vi "FTW-Tag-Core_Initialize.vi"(0 "Initialization Sequence":string, 5 "FTW Actor Instance Configuration":string, 11 "error in (no error)":errorcluster) -> (4 "FTW-Tag-Core Out":refnum<class "FTW-Tag-Core.lvclass">, 6 "Event Refnums":T1, 15 "error out":errorcluster)   [LabVIEW 2015, in "FTW-Tag-Core.lvclass"]
uses:
  FTW-Tag-Core.lvclass
  Message/Request/FTW-Message-IncomingRequest.lvclass
  Message/Base/FTW-Message.lvclass
  FTW-Tag-Core.lvclass/FTW-Tag-Core.ctl
  JSON/core/FTW-JSON-Core-EncodingFlags.vi
  JSON/FTW-JSON-Parse.vi
  Reflection/FTW-Reflection-Type.vi
  CodeGen/JSON Deserialize/FTW-JSON-Core-GetFlattenedValue.vi
  CodeGen/JSON Deserialize/FTW-JSON-Deserialize.xnode
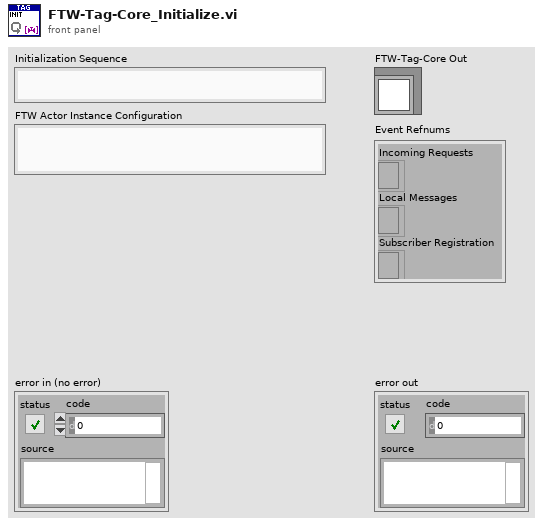
[diagram p1: front panel]
types:
  T1 = cluster{"Incoming Requests":refnum<event-registration>, "Local Messages":refnum<event-registration>, "Subscriber Registration":refnum<event-registration>}
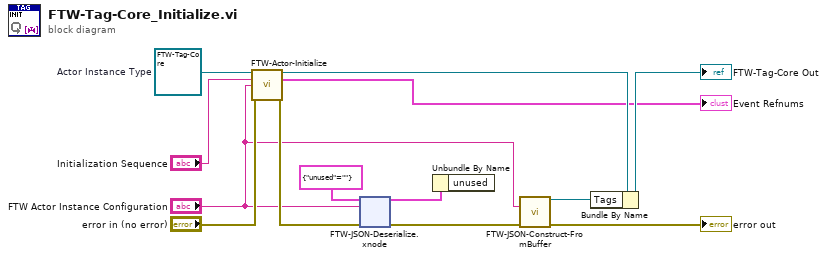
[diagram p0: block diagram]
diagram:
  w13 = refnum<class "FTW-Tag-Core.lvclass"> refnum  # Actor Instance Type
  n1 = call-dynamic "FTW-Actor-Initialize.vi"("FTW Actor Instance Type"=w13, "Initialization Job Sequence"="Initialization Sequence", "Actor Instance Configuration"="FTW Actor Instance Configuration", "error in"="error in (no error)") -> ("FTW Actor Instance"=w8:refnum<class "FTW-Tag-Core.lvclass">, "Event Refnums"=→"Event Refnums":T1, "error out"=w6:errorcluster)  [unwired: 9 in]
  n2 = xnode "FTW-JSON-Deserialize.xnode"("Type and Defaults"=cluster{"unused":string} {"unused"=""}, "JSON String"="FTW Actor Instance Configuration", "error in"=w6) -> ("Values"=w9:cluster{"unused":string}, "error out"=w11:errorcluster)
  n3 = Unbundle By Name(w9) -> ()  [unwired: 1 out]
  n4 = call "FTW-JSON-Construct-FromBuffer.vi"("JSON String (UTF-8)"="FTW Actor Instance Configuration", "error in"=w11) -> ("JSON"=w2:refnum<class "FTW-Container.lvclass">, "error out"=→"error out":errorcluster)  [unwired: 12 in]
  n5 = Bundle By Name(cluster=w8, "Tags"=w2) -> (→"FTW-Tag-Core Out":refnum<class "FTW-Tag-Core.lvclass">)
